vi "Search for Match.vi"(8 "dy":sgl, 9 "dx":sgl, 10 "Match":T1 {"Bounding Box"."y" format="%.2f"; "Bounding Box"."x" format="%.2f"; "Position"."y" format="%.2f"; "Position"."x" format="%.2f"; "Score" format="%.2f"; "Scale" format="%.2f"; "Angle" format="%.2f"}, 11 "Matches":T2(array[cluster]) {"Bounding Box"."y" format="%.2f"; "Bounding Box"."x" format="%.2f"; "Position"."y" format="%.2f"; "Position"."x" format="%.2f"; "Score" format="%.2f"; "Scale" format="%.2f"; "Angle" format="%.2f"}) -> (1 "Existing Match":T1 {"Bounding Box"."y" format="%.2f"; "Bounding Box"."x" format="%.2f"; "Position"."y" format="%.2f"; "Position"."x" format="%.2f"; "Score" format="%.2f"; "Scale" format="%.2f"; "Angle" format="%.2f"}, 2 "Match (duplicate)":T1 {"Bounding Box"."y" format="%.2f"; "Bounding Box"."x" format="%.2f"; "Position"."y" format="%.2f"; "Position"."x" format="%.2f"; "Score" format="%.2f"; "Scale" format="%.2f"; "Angle" format="%.2f"}, 3 "Match in Matches?":bool)   [LabVIEW 2013]
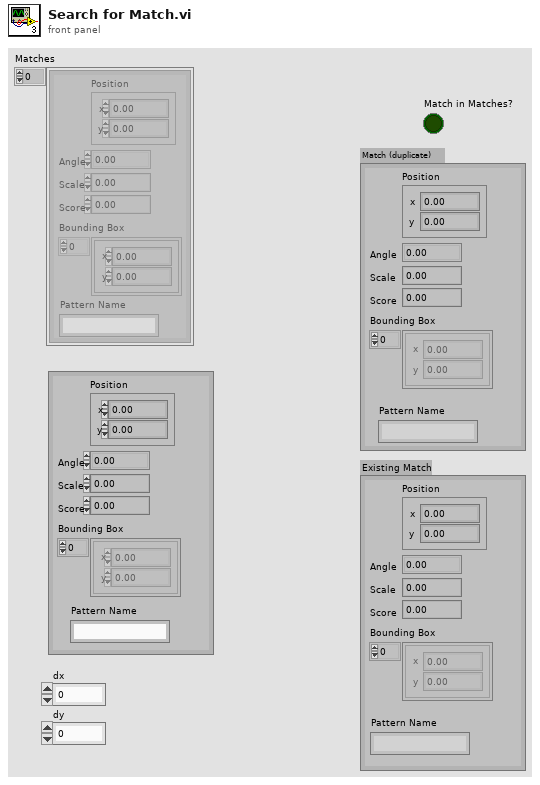
[diagram p1: front panel]
types:
  T1 = cluster{"Position":cluster{"x":sgl, "y":sgl}, "Angle":sgl, "Scale":sgl, "Score":sgl, "Bounding Box":cluster{"x":sgl, "y":sgl}[], "Pattern Name":string}
  T2 = cluster{"Position":cluster{"x":sgl, "y":sgl}, "Angle":sgl, "Scale":sgl, "Score":sgl, "Bounding Box":cluster{"x":sgl, "y":sgl}[], "Pattern Name":string}[]
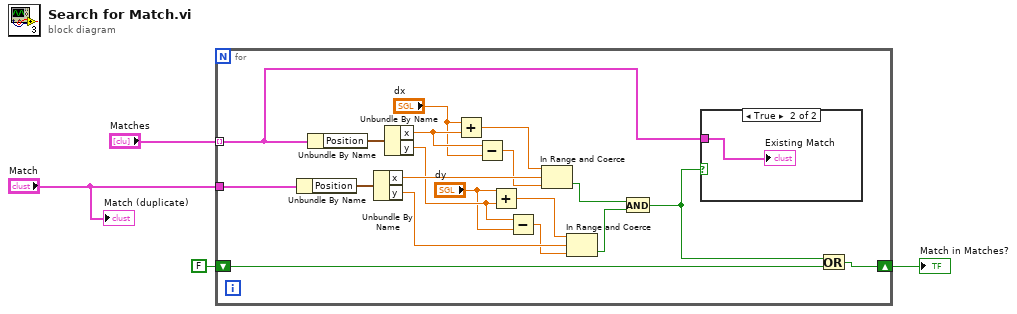
[diagram p0: block diagram]
diagram:
  n1 = for {
    tunnel: "Matches" -> [w5] mode=indexing
    tunnel: "Match" -> [w13]
    shift-right: [w12] -> w2
    shift-left: FALSE -> [w11]
    n2 = Unbundle By Name(w13) -> ("Position"=w22:cluster{"x":sgl, "y":sgl})
    n3 = Unbundle By Name(w5) -> ("Position"=w23:cluster{"x":sgl, "y":sgl})
    n4 = Unbundle By Name(w22) -> ("x"=w21:sgl, "y"=w20:sgl)
    n5 = Unbundle By Name(w23) -> ("x"=w19:sgl, "y"=w16:sgl)
    n6 = Add(x="dx", y=w19) -> (x+y=w18:sgl)
    n7 = Subtract(x=w19, y="dx") -> (x-y=w17:sgl)
    n8 = Add(x="dy", y=w16) -> (x+y=w15:sgl)
    n9 = Subtract(x=w16, y="dy") -> (x-y=w14:sgl)
    n10 = In Range and Coerce(upper limit=w18, x=w21, lower limit=w17) -> (In Range?=w10:bool)  [unwired: 1 out]
    n11 = In Range and Coerce(upper limit=w15, x=w20, lower limit=w14) -> (In Range?=w9:bool)  [unwired: 1 out]
    n12 = And(x=w10, y=w9) -> (x .and. y?=w6:bool)
    n13 = case shown="True" w6 {
      tunnel: w5 -> [_ w24]
      frame False {
      }
      frame True {
        "Existing Match" <- w24
      }
    }
    n14 = Or(x=w6, y=w11) -> (x .or. y?=w12:bool)
  }
  "Match in Matches?" <- w2
  "Match (duplicate)" <- "Match"
